vi "AI_wydobadz aktywne.vi"(8 "error in (no error)":errorcluster, 11 "AI param array in":T1[](array[typedef]) {"Numer" min=1 max=8 step=1}) -> (0 "error out":errorcluster, 2 "AI param aktywne out":T1[](array[typedef]) {"Numer" min=1 max=8 step=1}, 3 "Aktywne Array out":bool[](array[boolean]))   [LabVIEW 2013]
uses:
  Kontrolki/GUI/AI_parametry.ctl
  Kontrolki/GUI/AI_wartosc.ctl
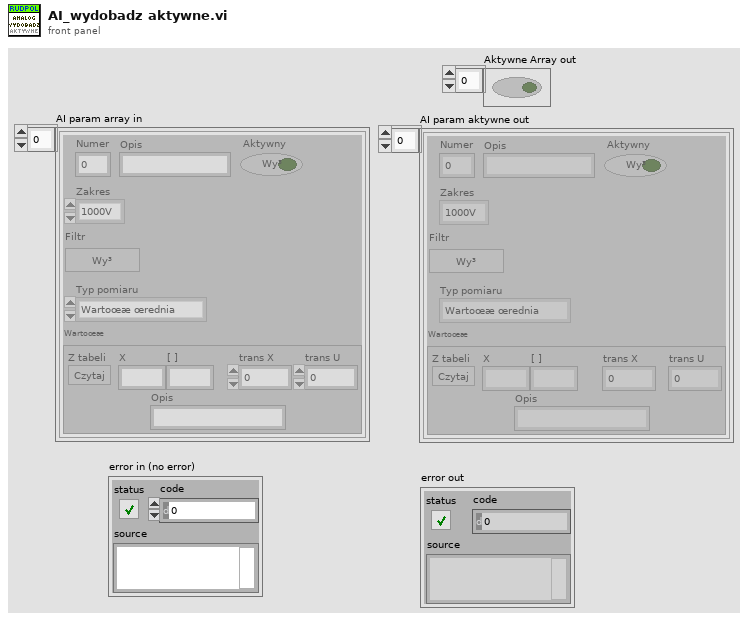
[diagram p1: front panel]
types:
  T1 = typedef "AI_parametry.ctl" = cluster{"Numer":u8, "Opis":string, "Zakres":enum16{"1000V", "300V", "30V", "3V", "0,3V"}, "Filtr":bool, "Typ pomiaru":enum16{"Wartoœæ œrednia", "Œrednia wyprostowana", "Wartoœæ skuteczna"}, "Aktywny":bool, "Wartoœæ":T2}
  T2 = typedef "AI_wartosc.ctl" = cluster{"X":string, "[ ]":string, "trans X":dbl, "trans U":dbl, "Z tabeli":bool, "Opis":string}
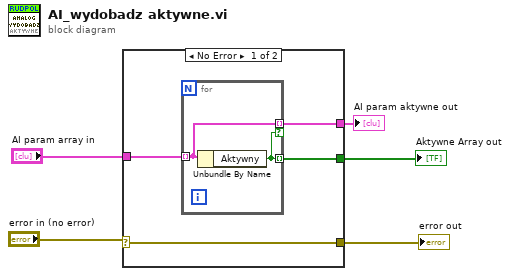
[diagram p0: block diagram]
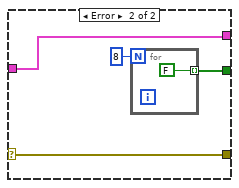
[diagram p2: hidden frame]
diagram:
  n1 = case shown="No Error" "error in (no error)" {
    selector: "error in (no error)" -> [w7 w15]
    tunnel: "AI param array in" -> [w9 w12]
    tunnel: [w8 w14] -> w4
    tunnel: [w7 w15] -> w2
    tunnel: [w6 w12] -> w1
    frame No Error {
      n2 = for {
        tunnel: w9 -> [w11] mode=indexing
        tunnel: [w10] -> w8 mode=indexing
        tunnel: [w11] -> w6 mode=indexing if=w10
        n3 = Unbundle By Name(w11) -> ("Aktywny"=w10:bool)
      }
    }
    frame Error {
      n4 = for {
        N: 8 -> [_]
        tunnel: [FALSE] -> w14 mode=indexing
      }
    }
  }
  "Aktywne Array out" <- w4
  "error out" <- w2
  "AI param aktywne out" <- w1
